vi "update config.vi"(8 "error in (no error)":errorcluster, 10 "user configurations":T2={"vst_device"=["VST_1", "VST_2"], "RF gain "=10.0, "buffer size"=524288, "center frequency (Hz) "=1000000000.0, "P2P sample rate"=200000000.0, "mode"=enum."5785 - 2*180MHz", "devicess"=["IF_transiver_0", "IF_transiver_1", "IF_transiver_2"], "file paths"=[path "C:/Users/PXIe8108_Demo/Documents/CHAIM DATA/chaim/5785_sync_for_elbit/data/pdw_test_file.tdms", path "C:/Users/PXIe8108_Demo/Documents/CHAIM DATA/chaim/5785_sync_for_elbit/data/pdw_test_file_1.tdms", path "C:/Users/PXIe8108_Demo/Documents/CHAIM DATA/chaim/5785_sync_for_elbit/data/pdw_test_file_2.tdms", path "C:/Users/PXIe8108_Demo/Documents/CHAIM DATA/chaim/5785_sync_for_elbit/data/pdw_test_file_3.tdms", path "C:/Users/PXIe8108_Demo/Documents/CHAIM DATA/chaim/5785_sync_for_elbit/data/pdw_test_file_4.tdms"], "gen for df"=FALSE}, 11 "p2p vst in":refnum<class "p2p vst.lvclass">) -> (0 "error out":errorcluster, 1 "min frequency":dbl, 2 "max frequency":dbl, 3 "p2p vst out":refnum<class "p2p vst.lvclass">)   [LabVIEW 2021, in "p2p vst.lvclass"]
uses:
  p2p vst.lvclass
  <vilib>/userdefined/High Color/nirio_resource_hc.ctl
  p2p vst.lvclass/p2p vst.ctl
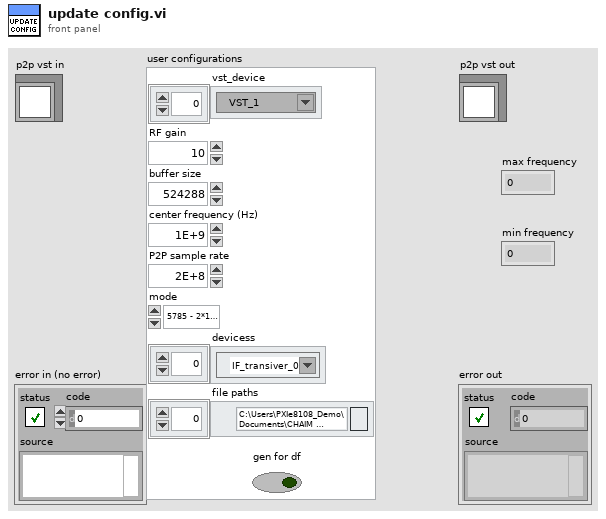
[diagram p1: front panel]
types:
  T1 = typedef "nirio_resource_hc.ctl" = tag
  T2 = cluster{"vst_device":refnum<k15>[], "RF gain ":dbl, "buffer size":u32, "center frequency (Hz) ":dbl, "P2P sample rate":dbl, "mode":enum16{"USRP - 180MHz", "5785 - 2*180MHz", "5785 - 3.2GHz", "P2P - VST"}, "devicess":T1[], "file paths":path[], "gen for df":bool}
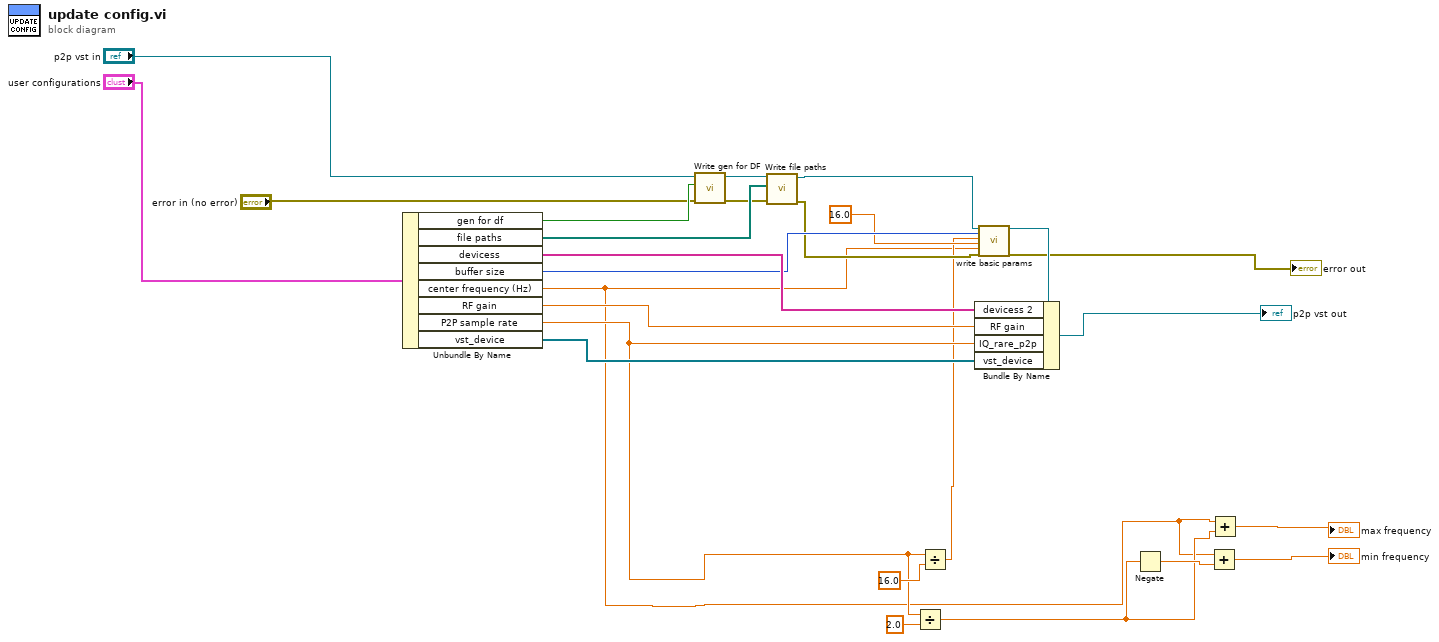
[diagram p0: block diagram]
diagram:
  n1 = Unbundle By Name("user configurations") -> ("gen for df"=w19:bool, "file paths"=w22:path[], "devicess"=w26:T1[], "buffer size"=w25:u32, "center frequency (Hz)"=w1:dbl, "RF gain"=w16:dbl, "P2P sample rate"=w4:dbl, "vst_device"=w10:refnum<k15>[])
  n2 = call-dynamic "Write gen for DF.vi"("error in (no error)"="error in (no error)", "gen for DF"=w19, "device_type in"="p2p vst in") -> ("error out"=w18:errorcluster, "device_type out"=w20:refnum<class "p2p vst.lvclass">)  [unwired: 7 in]
  n3 = call-dynamic "Write file paths.vi"("error in (no error)"=w18, "file paths"=w22, "device_type in"=w20) -> ("error out"=w17:errorcluster, "device_type out"=w21:refnum<class "p2p vst.lvclass">)  [unwired: 7 in]
  n4 = Divide(x=w4, y=2.0) -> (x/y=w8:dbl)
  n5 = Divide(x=w4, y=16.0 ("Fs  FPGA")) -> (x/y=w2:dbl)
  n6 = call-dynamic "write basic params.vi"("device_type in"=w21, "buffer size"=w25, "Fs  FPGA"=w2, "SPC"=16.0 ("Fs  FPGA"), "center frequency (Hz)"=w1, "error in (no error)"=w17) -> ("device_type out"=w23:refnum<class "p2p vst.lvclass">, "error out"=→"error out":errorcluster)  [unwired: 12 in]
  n7 = Bundle By Name(cluster=w23, "devicess 2"=w26, "RF gain"=w16, "IQ_rare_p2p"=w4, "vst_device"=w10) -> (→"p2p vst out":refnum<class "p2p vst.lvclass">)
  n8 = Negate(x=w8) -> (-x=w9:dbl)
  n9 = Add(x=w1, y=w9) -> (x+y=→"min frequency":dbl)
  n10 = Add(x=w1, y=w8) -> (x+y=→"max frequency":dbl)
